vi "PT1000 Data.vi"(10 "Resistance (Ohms)":dbl) -> (2 "Temperature (DegC)":dbl)   [LabVIEW 2010]
uses:
  <vilib>/Analysis/polynomials.llb/Scalar Polynomial Evaluation (DBL).vi
  <vilib>/Analysis/NI_AALPro.lvlib
panel:
  out "PolyCoefs":dbl[](array[numeric])
  out "Resistances":dbl[](array[numeric])
  out "Temps":dbl[](array[numeric])
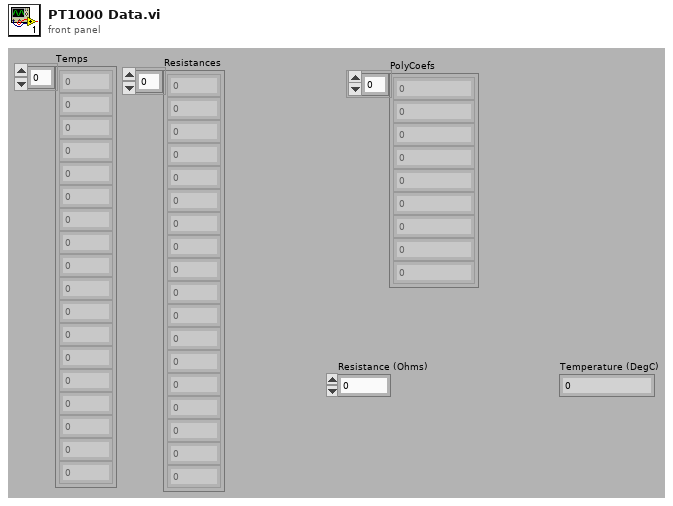
[diagram p1: front panel]
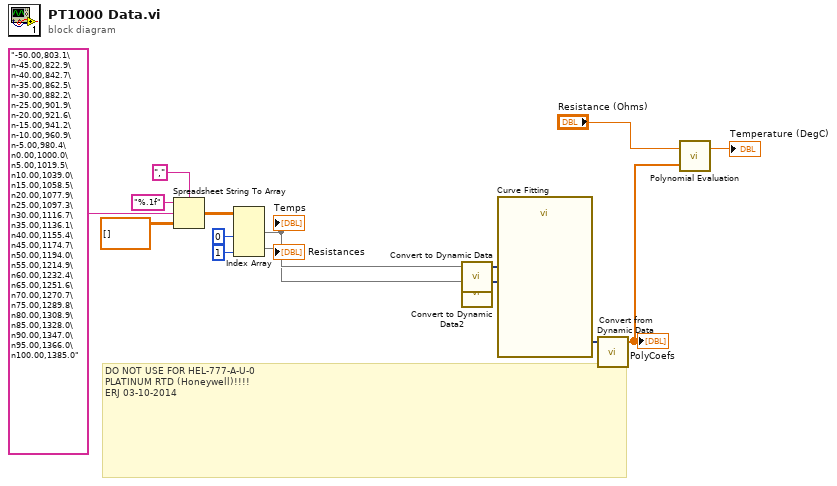
[diagram p0: block diagram]
diagram:
  # "DO NOT USE FOR HEL-777-A-U-0\nPLATINUM RTD (Honeywell)!!!!\nERJ 03-10-2014"
  n1 = Spreadsheet String To Array(delimiter (Tab)=",", format string="%.1f", spreadsheet string="-50.00,803.1\n-45.00,822.9\n-40.00,842.7\n-35.00,862.5\n-30.00,882.2\n-25.00,901.9\n-20.00,921.6\n-15.00,941.2\n-10.00,960.9\n-5.00,980.4\n0.00,1000.0\n5.00,1019.5\n10.00,1039.0\n15.00,1058.5\n20.00,1077.9\n25.00,1097.3\n30.00,1116.7\n35.00,1136.1\n40.00,1155.4\n45.00,1174.7\n50.00,1194.0\n55.00,1214.9\n60.00,1232.4\n65.00,1251.6\n70.00,1270.7\n75.00,1289.8\n80.00,1308.9\n85.00,1328.0\n90.00,1347.0\n95.00,1366.0\n100.00,1385.0", array type (2D Dbl)=dbl[][] []) -> (array=w11:dbl[][])
  n2 = Index Array(array=w11, index (col) #1=0 ("disabled index (col)"), index (col) #2=1 ("index (col)")) -> (element #1=w5:dbl[], element #2=w4:dbl[])  [unwired: 2 in]
  "Temps" <- w5
  "Resistances" <- w4
  n3 = call "Convert to Dynamic Data"("Array"=w5) -> ("Dynamic Data Type"=w8:dynamicdata)  [unwired: 3 in]
  n4 = call "Convert to Dynamic Data2"("Array"=w4) -> ("Dynamic Data Type"=w7:dynamicdata)  [unwired: 3 in]
  n5 = call "Curve Fitting"("Locations"=w7, "Signals"=w8) -> ("polynomial coefficients"=w6:dynamicdata)  [unwired: 5 in, 4 out]
  n6 = call "Convert from Dynamic Data"("Dynamic Data Type"=w6) -> ("Array"=w1:dbl[])  [unwired: 3 in]
  "PolyCoefs" <- w1
  n7 = call-poly <vilib>:"Polynomial Evaluation.vi"("P(x)"=w1, "a"="Resistance (Ohms)") -> ("P(a)"=→"Temperature (DegC)":dbl)  [unwired: 1 out]
